vi "Period to RPM.vi"(10 "Period (sec)":dbl) -> (2 "RPM":dbl)   [LabVIEW 2012]
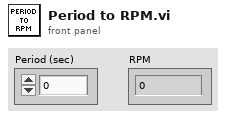
[diagram p1: front panel]
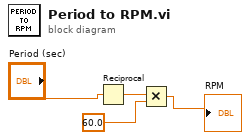
[diagram p0: block diagram]
diagram:
  n1 = Reciprocal(x="Period (sec)") -> (1/x=w1:dbl)
  n2 = Multiply(x=w1, y=60.0) -> (x*y=→"RPM":dbl)
